vi "rhoplus.vi"(10 "Array 3":dbl[](array[numeric]), 11 "Array in":dbl[](array[numeric])) -> (3 "Array out":dbl[](array[numeric]))   [LabVIEW 2019]
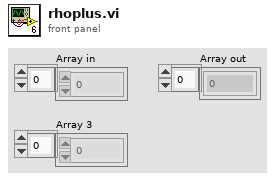
[diagram p1: front panel]
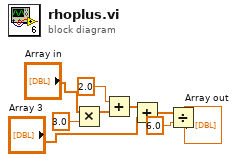
[diagram p0: block diagram]
diagram:
  n1 = Multiply(x="Array in", y=3.0) -> (x*y=w2:dbl[])
  n2 = Add(x=2.0, y=w2) -> (x+y=w4:dbl[])
  n3 = Add(x=w4, y="Array 3") -> (x+y=w5:dbl[])
  n4 = Divide(x=w5, y=6.0) -> (x/y=→"Array out":dbl[])
